vi "PalmSense Message Loop.vi"(8 "error in (no error)":errorcluster) -> (0 "error out":errorcluster)   [LabVIEW 2020, in "PalmSens.lvlib"]
doc: "Message loop for handling messages pertaining to the acquisition of data from the hardware."
uses:
  PalmSens.lvlib
  <instrlib>/PalmSens SDK for LabVIEW 5.10/PalmSens/PalmSens.lvclass
  support/PCT FGV CMD.ctl
  Acquisition State.ctl
  PalmSense Hardware Configuration.ctl
  support/Message Queue/Message Cluster.ctl
  support/Message Queue/Enqueue Message (Single).vi
  <vilib>/Utility/error.llb/Error Cluster From Error Code.vi
  <vilib>/ErrorRing/Error Ring.xnode
  support/Message Queue/Message Queue.lvlib
panel:
  in  "PalmSens.lvclass":refnum<class "PalmSens.lvclass">
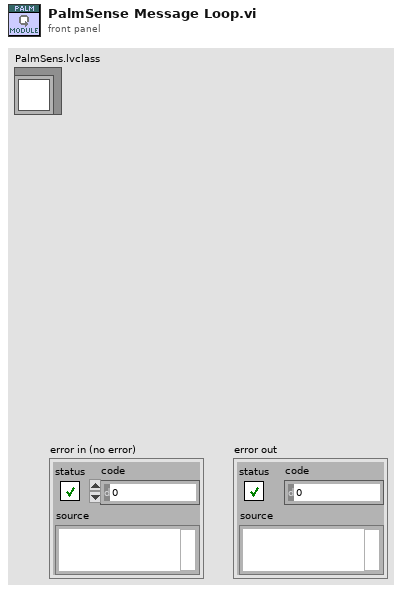
[diagram p1: front panel]
types:
  T1 = typedef "PCT FGV CMD.ctl" = enum16{"INIT", "GET", "SET"}
  T2 = typedef "Message Queue.lvlib/All Message Queues.ctl" = cluster{"UI":refnum<queue>, "Logging":refnum<queue>, "LOG":refnum<queue>, "ALARM":refnum<queue>, "Test":refnum<queue>, "Answer":refnum<queue>, "PLC":refnum<queue>, "DB":refnum<queue>, "Report":refnum<queue>, "OPC":refnum<queue>, "Procedure":refnum<queue>, "PalmSens":refnum<queue>, "SYS 7000 Reader":refnum<queue>, "SWITCH":refnum<queue>, "MOTOR":refnum<queue>, "MOTION":refnum<queue>, "HIDEN":refnum<queue>, "VALVE":refnum<queue>, "MFC":refnum<queue>, "PUMP IN":refnum<queue>, "PUMP OUT":refnum<queue>}
  T3 = typedef "PalmSens.lvlib/PalmSense Hardware Configuration.ctl" = cluster{"PalmSens.lvclass":refnum<class "PalmSens.lvclass">, "Writer Queue":refnum<queue>, "Enable":bool, "Is Measuring Ref":refnum<vi>, "Method":cluster{"Name":string, "Method Ref":variant}, "PS Live Curve Result":refnum<vi>}
  T4 = typedef "Message Queue.lvlib/Message Cluster.ctl" = cluster{"Message":string, "Message Data":variant}
  T5 = typedef "PalmSens.lvlib/Acquisition State.ctl" = enum16{"Idle", "Initialized"}
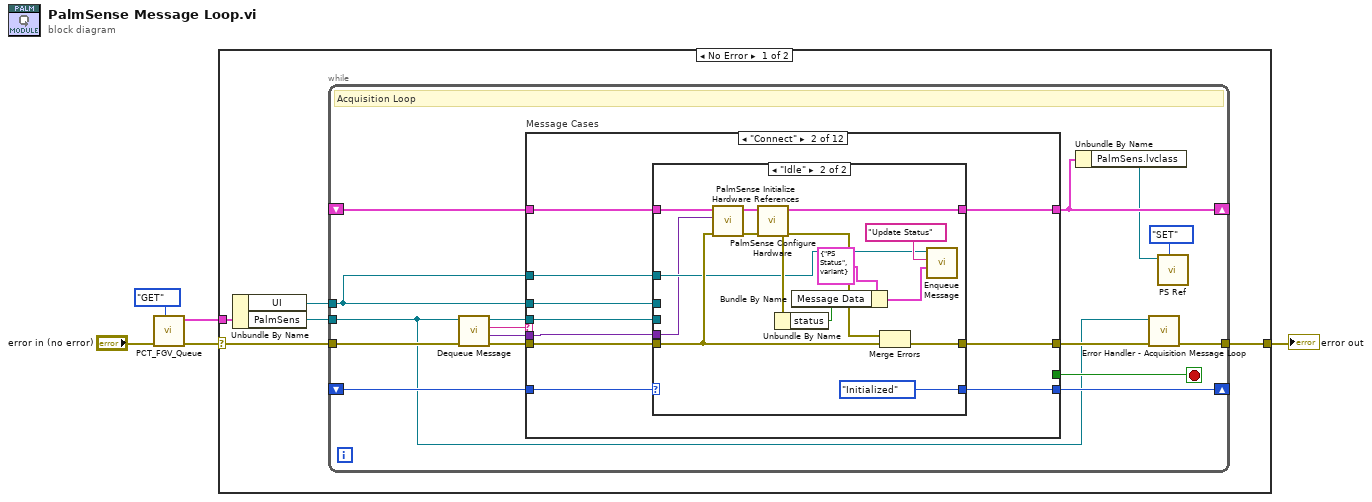
[diagram p0: block diagram]
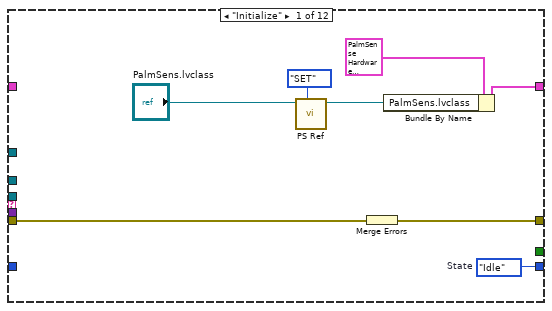
[diagram p2: hidden frame]
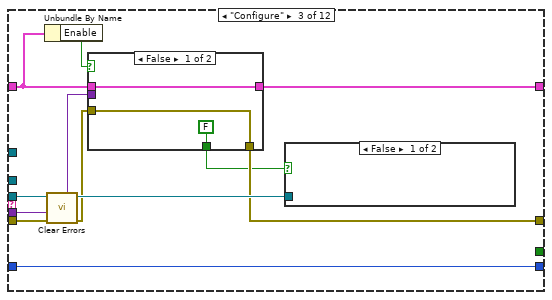
[diagram p4: hidden frame]
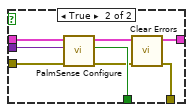
[diagram p5: hidden frame]
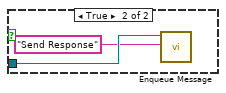
[diagram p6: hidden frame]
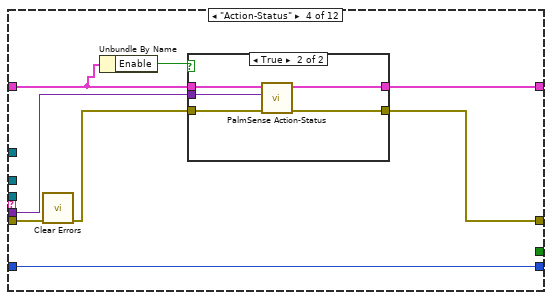
[diagram p7: hidden frame]
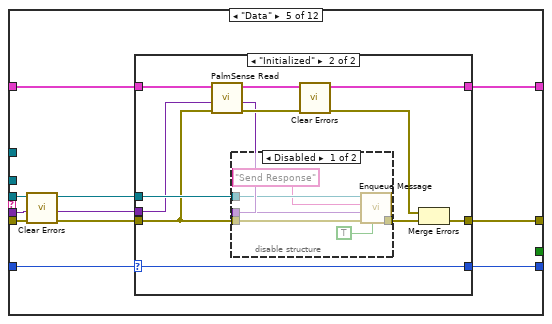
[diagram p9: hidden frame]
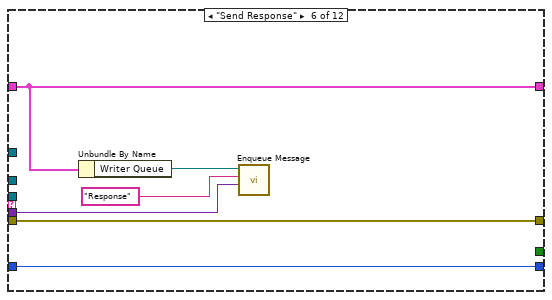
[diagram p12: hidden frame]
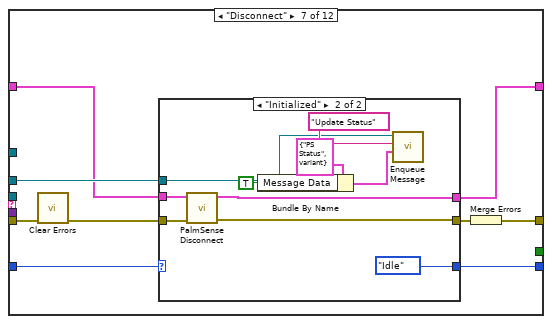
[diagram p13: hidden frame]
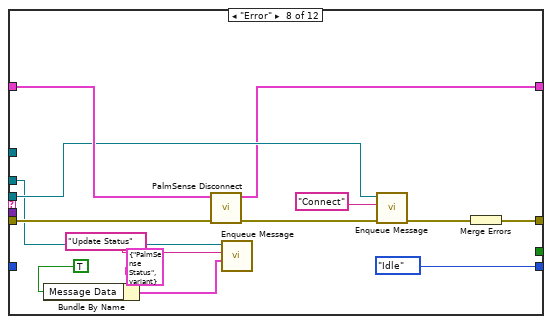
[diagram p15: hidden frame]
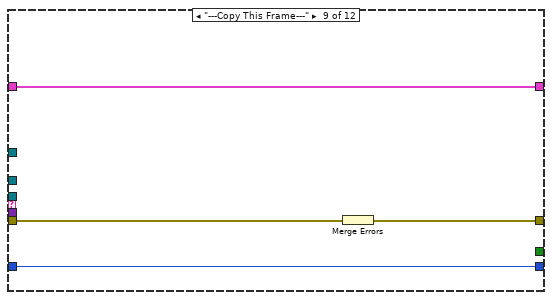
[diagram p16: hidden frame]
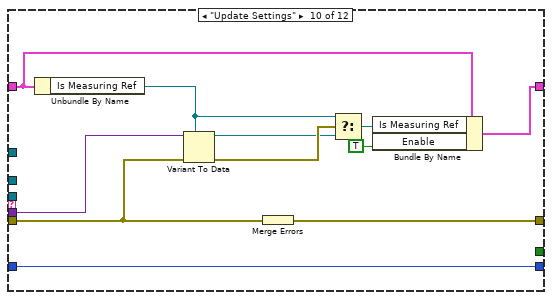
[diagram p17: hidden frame]
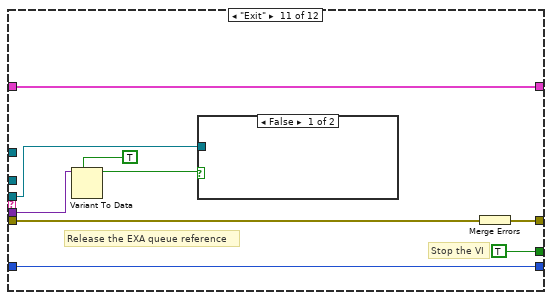
[diagram p18: hidden frame]
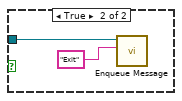
[diagram p19: hidden frame]
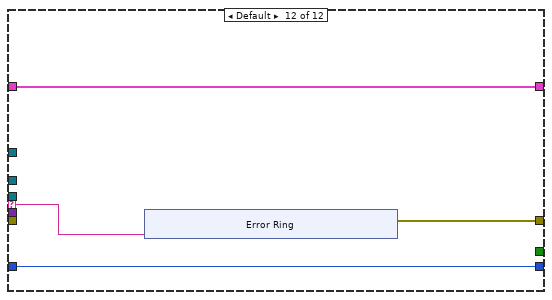
[diagram p20: hidden frame]
diagram:
  n1 = call "PCT_FGV_Queue.vi"("CMD"=PCT_FGV_CMD."GET", "error in (no error)"="error in (no error)") -> ("error out"=w3:errorcluster, "Message Queues out"=w2:T2)  [unwired: 8 in]
  n2 = case shown="No Error" w3 {
    selector: w3 -> [w7 w207]
    tunnel: w2 -> [w10 _]
    tunnel: [w8 w207] -> w5
    frame No Error {
      n3 = Unbundle By Name(w10) -> ("UI"=w6:refnum<queue>, "PalmSens"=w9:refnum<queue>)
      n4 = while {
        tunnel: w9 -> [w14]
        shift-right: [w12] -> _
        shift-left: _ -> [w26]
        tunnel: w6 -> [w17]
        shift-right: [w20] -> _
        shift-left: _ -> [w21]
        tunnel: w7 -> [w24]
        tunnel: [w15] -> w8
        stop <- w25 stop-if-true
        # "Acquisition Loop"
        n5 = call "Dequeue Message.vi"("error in (no error)"=w24, "Message Queue"=w14) -> ("error out"=w23:errorcluster, "Message Data"=w22:variant, "Message"=w18:string, "dup Message Queue"=w19:refnum<queue>)  [unwired: 6 in]
        n6 = case "Message Cases" shown="\"Connect\"" w18 {
          selector: w18 -> [_ _ _ _ _ _ _ _ _ _ _ w196]
          tunnel: w19 -> [_ w36 w67 _ w106 _ _ w162 _ _ w187 _]
          tunnel: w23 -> [w33 w42 w69 w88 w105 w128 w141 w168 w173 w180 w186 _]
          tunnel: [w34 w44 w66 w87 w107 w128 w142 w169 w171 w184 w192 w197] -> w16
          tunnel: w26 -> [_ w43 w63 w85 w103 w130 w134 w166 w172 w175 w191 w199]
          tunnel: [w30 w41 w68 w89 w104 w130 w135 w156 w172 w176 w191 w199] -> w12
          tunnel: [_ _ _ _ _ _ _ _ _ _ TRUE _] -> w25
          tunnel: w22 -> [_ w35 w70 w90 w100 w131 _ _ _ w183 w185 _]
          tunnel: w17 -> [_ w38 _ _ _ _ w137 w158 _ _ _ _]
          tunnel: w21 -> [_ w39 w71 w91 w101 w132 w139 _ w170 w179 w190 w198]
          tunnel: [w32 w40 w71 w91 w102 w132 w138 Acquisition_State."Idle" ("State") w170 w179 w190 w198] -> w20
          tunnel: w17 -> [_ w37 _ _ _ _ _ _ _ _ _ _]
          frame "Initialize" {
            w32 = Acquisition_State."Idle"  # State
            # "Initialize  - Initialize is currently a no-op.  The hardware initialization takes place in the 'Start' message."
            n7 = call "PS Ref.vi"("CMD"=PCT_FGV_CMD."SET", "PalmSens.lvclass"="PalmSens.lvclass") -> ("PalmSens.lvclass out"=w27:refnum<class "PalmSens.lvclass">)  [unwired: 8 in, 1 out]
            n8 = Merge Errors(w33) -> (w34:errorcluster)
            n9 = Bundle By Name(cluster=T3 {"PalmSens.lvclass"=refnum, "Writer Queue"=refnum, "Enable"=FALSE, "Is Measuring Ref"=refnum, "Method"={"Name"="", "Method Ref"=variant}, "PS Live Curve Result"=refnum} ("Data Cluster"), "PalmSens.lvclass"=w27) -> (w30:T3)
          }
          frame "Connect" {
            # "Start - Configure and start the acquisition."
            n10 = case shown="\"Idle\"" w39 {
              selector: w39 -> [w45 _]
              tunnel: [w46 w61] -> w44
              tunnel: w43 -> [w47 w60]
              tunnel: w42 -> [w46 w56]
              tunnel: w36 -> [_ _]
              tunnel: [w47 w58] -> w41
              tunnel: [w45 Acquisition_State."Initialized" ("Acquisition State")] -> w40
              tunnel: w38 -> [_ _]
              tunnel: w37 -> [_ w50]
              tunnel: w35 -> [_ w48]
              frame "Initialized" {
                # "The system is already acquiring. Ignore the \"Start\" message."
              }
              frame "Idle" {
                # "If the system is idle, start the acquisition."
                n11 = call "PalmSense Initialize Hardware References.vi"("error in (no error)"=w56, "Data"=w48, "Hardware Resources in"=w60) -> ("error out"=w54:errorcluster, "Hardware Resources out"=w55:T3)  [unwired: 7 in]
                n12 = call "PalmSense Configure Hardware.vi"("error in (no error)"=w54, "Hardware Resources in"=w55) -> ("error out"=w59:errorcluster, "Hardware Resources out"=w58:T3)  [unwired: 8 in]
                n13 = Unbundle By Name(w54) -> ("status"=w49:bool)
                n14 = Bundle By Name(cluster=T4 {"Message"="PS Status", "Message Data"=variant} ("Message Cluster"), "Message Data"=w49) -> (w53:T4)
                n15 = Merge Errors(w59, w56) -> (w61:errorcluster)
                n16 = call-poly "Enqueue Message.vi"("Message Data"=w53, "Message"="Update Status", "Message Queue"=w50) -> ()  [unwired: 7 in, 2 out]
              }
            }
          }
          frame "Configure" {
            # "Start - Configure and start the acquisition."
            n17 = Unbundle By Name(w63) -> ("Enable"=w62:bool)
            n18 = call <vilib>:"Clear Errors.vi"("error in (no error)"=w69) -> ("error out"=w64:errorcluster)  [unwired: 5 in, 1 out]
            n19 = case shown="False" w62 {
              tunnel: w70 -> [_ w75]
              tunnel: w63 -> [w74 w81]
              tunnel: [w74 w80] -> w68
              tunnel: [w72 w79] -> w66
              tunnel: [FALSE ("Send Resp") w78] -> w65
              tunnel: w64 -> [w72 w77]
              frame False {
              }
              frame True {
                n20 = call "PalmSense Configure.vi"("error in (no error)"=w77, "Message Data"=w75, "Data Cluster"=w81) -> ("error out"=w76:errorcluster, "Send Resp"=w78:bool, "Data Cluster out"=w80:T3)  [unwired: 6 in]
                n21 = call <vilib>:"Clear Errors.vi"("error in (no error)"=w76) -> ("error out"=w79:errorcluster)  [unwired: 5 in, 1 out]
              }
            }
            n22 = case shown="False" w65 {
              tunnel: w67 -> [_ w83]
              frame False {
              }
              frame True {
                n23 = call-poly "Enqueue Message.vi"("Message"="Send Response", "Message Queue"=w83) -> ()  [unwired: 8 in, 2 out]
              }
            }
          }
          frame "Action-Status" {
            # "Start - Configure and start the acquisition."
            n24 = call <vilib>:"Clear Errors.vi"("error in (no error)"=w88) -> ("error out"=w86:errorcluster)  [unwired: 5 in, 1 out]
            n25 = Unbundle By Name(w85) -> ("Enable"=w84:bool)
            n26 = case shown="True" w84 {
              tunnel: w90 -> [_ w98]
              tunnel: [w93 w97] -> w89
              tunnel: w85 -> [w93 w96]
              tunnel: [w92 w95] -> w87
              tunnel: w86 -> [w92 w94]
              frame False {
              }
              frame True {
                n27 = call "PalmSense Action-Status.vi"("error in (no error)"=w94, "Message Data"=w98, "Data Cluster"=w96) -> ("error out"=w95:errorcluster, "Data Cluster out"=w97:T3)  [unwired: 7 in]
              }
            }
          }
          frame "Data" {
            # "Acquire - Acquire data from the hardware. Since this is a continuous acquisition, this message will always message itself to run again."
            n28 = call <vilib>:"Clear Errors.vi"("error in (no error)"=w105) -> ("error out"=w99:errorcluster)  [unwired: 5 in, 1 out]
            n29 = case shown="\"Initialized\"" w101 {
              selector: w101 -> [w108 w115]
              tunnel: [w109 w121] -> w107
              tunnel: w106 -> [_ w119]
              tunnel: w99 -> [w109 w114]
              tunnel: [w110 w117] -> w104
              tunnel: w103 -> [w110 w116]
              tunnel: [w108 w115] -> w102
              tunnel: w100 -> [_ w113]
              frame "Idle" {
              }
              frame "Initialized" {
                # "Read  data"
                n30 = call "PalmSense Read.vi"("error in (no error)"=w114, "Message Data"=w113, "Hardware Resources in"=w116) -> ("error out"=w118:errorcluster, "Message Data Out"=w112:variant, "Hardware Resources out"=w117:T3)  [unwired: 6 in]
                n31 = disable-structure shown="Disabled" {
                  disable-tunnel: [w127 _] -> w120
                  disable-tunnel: w119 -> [w126 _]
                  disable-tunnel: w114 -> [w124 _]
                  disable-tunnel: w112 -> [w123 _]
                  frame Disabled {
                    n32 = call-poly "Enqueue Message.vi"("Priority Message? (F)"=TRUE, "error in (no error)"=w124, "Message Data"=w123, "Message"="Send Response", "Message Queue"=w126) -> ("error out"=w127:errorcluster)  [unwired: 5 in, 1 out]
                  }
                  frame Enabled {
                  }
                }
                n33 = call <vilib>:"Clear Errors.vi"("error in (no error)"=w118) -> ("error out"=w111:errorcluster)  [unwired: 5 in, 1 out]
                n34 = Merge Errors(w111, w120) -> (w121:errorcluster)
              }
            }
          }
          frame "Send Response" {
            # "Acquire - Acquire data from the hardware. Since this is a continuous acquisition, this message will always message itself to run again."
            n35 = Unbundle By Name(w130) -> ("Writer Queue"=w129:refnum<queue>)
            n36 = call-poly "Enqueue Message.vi"("Message Data"=w131, "Message"="Response", "Message Queue"=w129) -> ()  [unwired: 7 in, 2 out]
          }
          frame "Disconnect" {
            # "Stop - Stop the Acquisition."
            n37 = call <vilib>:"Clear Errors.vi"("error in (no error)"=w141) -> ("error out"=w136:errorcluster)  [unwired: 5 in, 1 out]
            n38 = case shown="\"Initialized\"" w139 {
              selector: w139 -> [w144 _]
              tunnel: w136 -> [w145 w155]
              tunnel: [w145 w154] -> w140
              tunnel: w134 -> [w143 w153]
              tunnel: [w144 Acquisition_State."Idle" ("State")] -> w138
              tunnel: w137 -> [_ w147]
              tunnel: [w143 w146] -> w135
              frame "Idle" {
                # "The system is already idle. Ignore the \"Stop\" message."
              }
              frame "Initialized" {
                # "If the system is acquiring, stop the acquisition."
                n39 = call "PalmSense Disconnect.vi"("error in (no error)"=w155, "Hardware Resources in"=w153) -> ("error out"=w154:errorcluster, "Hardware Resources out"=w146:T3)  [unwired: 8 in]
                n40 = Bundle By Name(cluster=T4 {"Message"="PS Status", "Message Data"=variant} ("Message Cluster"), "Message Data"=TRUE ("status")) -> (w151:T4)
                n41 = call-poly "Enqueue Message.vi"("Message Data"=w151, "Message"="Update Status", "Message Queue"=w147) -> ()  [unwired: 7 in, 2 out]
              }
            }
            n42 = Merge Errors(w140) -> (w142:errorcluster)
          }
          frame "Error" {
            # "Stop - Stop the Acquisition."
            n43 = Bundle By Name(cluster=T4 {"Message"="PalmSense Status", "Message Data"=variant} ("Message Cluster"), "Message Data"=TRUE) -> (w161:T4)
            n44 = call "PalmSense Disconnect.vi"("error in (no error)"=w168, "Hardware Resources in"=w166) -> ("error out"=w164:errorcluster, "Hardware Resources out"=w156:T3)  [unwired: 8 in]
            n45 = call-poly "Enqueue Message.vi"("Message Data"=w161, "Message"="Update Status", "Message Queue"=w158) -> ()  [unwired: 7 in, 2 out]
            n46 = call-poly "Enqueue Message.vi"("error in (no error)"=w164, "Message"="Connect", "Message Queue"=w162) -> ("error out"=w167:errorcluster)  [unwired: 7 in, 1 out]
            n47 = Merge Errors(w167) -> (w169:errorcluster)
          }
          frame "---Copy This Frame---" {
            # "Duplicate this frame when creating new messages.  Change this comment in the duplicated frame to describe this message."
            n48 = Merge Errors(w173) -> (w171:errorcluster)
          }
          frame "Update Settings" {
            # "New settings are available, update the current ones stored in the shift register with the settings sent as part of the message"
            n49 = Unbundle By Name(w175) -> ("Is Measuring Ref"=w177:refnum<vi>)
            n50 = Variant To Data(error in=w180, type=w177, Variant=w183) -> (data=w181:refnum<vi>, error out=w182:errorcluster)
            n51 = Merge Errors(w180) -> (w184:errorcluster)
            n52 = Select(t=w177, s=w182, f=w181) -> (s? t:f=w178:refnum<vi>)
            n53 = Bundle By Name(cluster=w175, "Is Measuring Ref"=w178, "Enable"=TRUE) -> (w176:T3)
          }
          frame "Exit" {
            # "Release the EXA queue reference"
            # "Stop the VI"
            # "Exit - Send the Exit message to the UI Message Handler."
            n54 = Variant To Data(type=TRUE, Variant=w185) -> (data=w189:bool)  [unwired: 1 in, 1 out]
            n55 = case shown="False" w189 {
              tunnel: w187 -> [_ w195]
              frame False {
              }
              frame True {
                n56 = call-poly "Enqueue Message.vi"("Message"="Exit", "Message Queue"=w195) -> ()  [unwired: 8 in, 2 out]
              }
            }
            n57 = Merge Errors(w186) -> (w192:errorcluster)
          }
          frame Default {
            # "'Default' case only runs if there is a message that isn't defined in any of the other cases.  Output a programming error."
            n58 = xnode "Error Ring"("parameter 0"=w196) -> ("error out"=w197:errorcluster)
          }
        }
        n59 = Unbundle By Name(w12) -> ("PalmSens.lvclass"=w11:refnum<class "PalmSens.lvclass">)
        n60 = call "Error Handler - Acquisition Message Loop.vi"("error in (no error)"=w16, "Message Queue"=w14) -> ("dup error in"=w15:errorcluster)  [unwired: 8 in, 1 out]
        n61 = call "PS Ref.vi"("CMD"=PCT_FGV_CMD."SET", "PalmSens.lvclass"=w11) -> ()  [unwired: 8 in, 2 out]
      }
    }
    frame Error {
    }
  }
  "error out" <- w5
